vi "max gen.vi"(10 "reset every":u32, 11 "raw sampels":i16[](array[numeric])=[0, 0, 0, 0]) -> (2 "max for time":i16, 3 "max of them":i16)   [LabVIEW 2021]
uses:
  <instrlib>/_niInstr/Basic Elements/v1/FPGA/Private/Count Up U32.vi
  <instrlib>/_niInstr/Basic Elements/v1/FPGA/niInstr Basic Elements v1 FPGA.lvlib
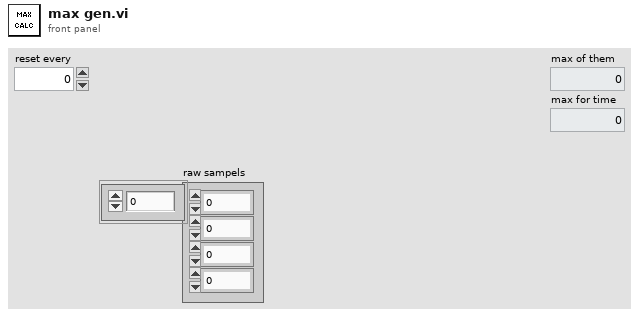
[diagram p1: front panel]
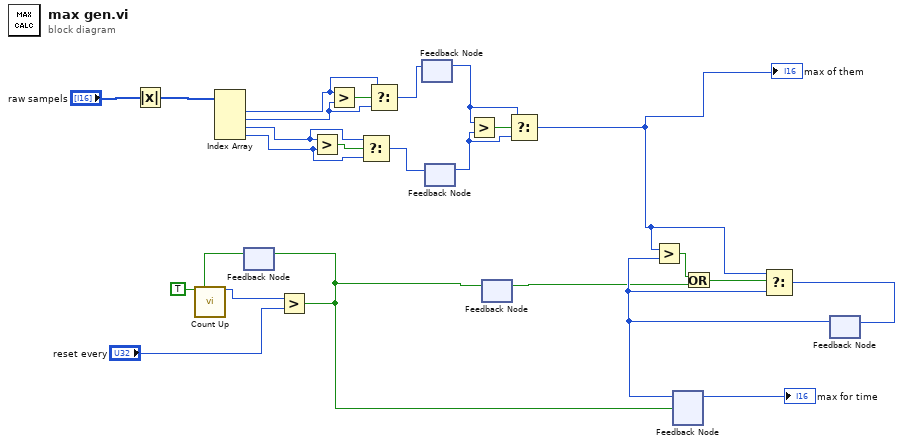
[diagram p0: block diagram]
diagram:
  n1 = Absolute Value(x="raw sampels") -> (abs(x)=w24:i16[])
  n2 = Index Array(array=w24) -> (element #1=w18:i16, element #2=w19:i16, element #3=w22:i16, element #4=w21:i16)  [unwired: 4 in]
  n3 = feedback #1() -> (w13:bool)  [unwired: 1 in]
  n4 = call-poly <instrlib>:"Count Up.vi"("increment"=TRUE, "reset"=w13) -> ("count out"=w15:u32)  [unwired: 13 in]
  n5 = Greater?(x=w15, y="reset every") -> (0:w2:bool)
  n6 = feedback-in #1(w2) -> ()
  n7 = Greater?(x=w22, y=w21) -> (0:w23:bool)
  n8 = Greater?(x=w18, y=w19) -> (0:w20:bool)
  n9 = Select(t=w22, s=w23, f=w21) -> (s? t:f=w6:i16)
  n10 = Select(t=w18, s=w20, f=w19) -> (s? t:f=w4:i16)
  n11 = feedback #2() -> (w3:i16)  [unwired: 1 in]
  n12 = feedback-in #2(w4) -> ()
  n13 = feedback-in #3(w6) -> ()
  n14 = feedback #3() -> (w5:i16)  [unwired: 1 in]
  n15 = Greater?(x=w3, y=w5) -> (0:w17:bool)
  n16 = feedback #4() -> (w1:bool)  [unwired: 1 in]
  n17 = feedback-in #4(w2) -> ()
  n18 = Select(t=w3, s=w17, f=w5) -> (s? t:f=w9:i16)
  "max of them" <- w9
  n19 = feedback #5() -> (→"max for time":i16)  [unwired: 1 in]
  n20 = feedback #6() -> (w8:i16)  [unwired: 1 in]
  n21 = Greater?(x=w9, y=w8) -> (0:w10:bool)
  n22 = feedback-in #5(w8, w2) -> ()
  n23 = Or(x=w10, y=w1) -> (x .or. y?=w11:bool)
  n24 = Select(t=w9, s=w11, f=w8) -> (s? t:f=w12:i16)
  n25 = feedback-in #6(w12) -> ()
